vi "Convert to TDMS.vi"(6 "Fiirst call":bool, 8 "Error In":errorcluster, 9 "Add to channel list":string, 10 "TDMS target file":path, 11 "DataPlugin source file":path) -> (0 "Error Out":errorcluster, 1 "channel name(s) out":string[](array[string]), 2 "group name out":string, 3 "File output":path)   [LabVIEW 2015]
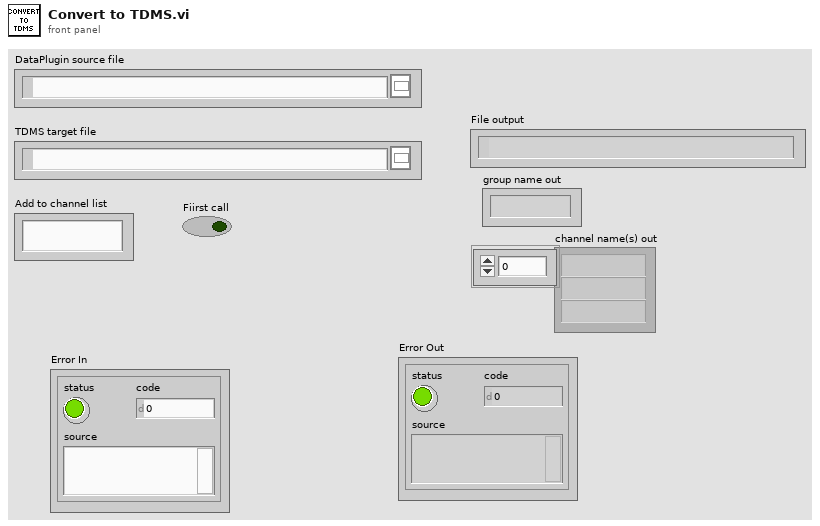
[diagram p1: front panel]
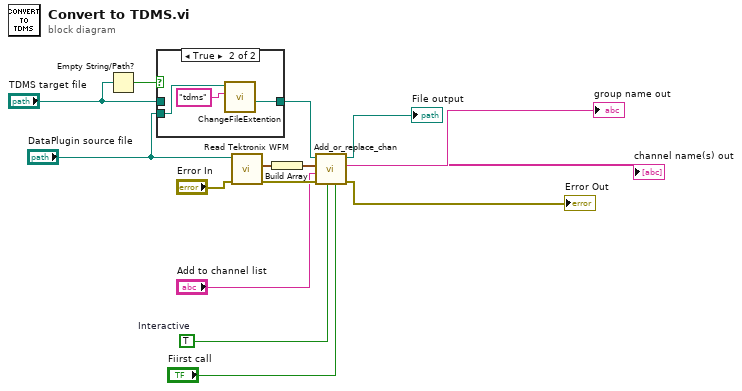
[diagram p0: block diagram]
diagram:
  w8 = TRUE  # Interactive
  n1 = Empty String/Path?(string/path="TDMS target file") -> (empty?=w11:bool)
  n2 = case shown="True" w11 {
    tunnel: "DataPlugin source file" -> [_ w18]
    tunnel: [w16 w17] -> w10
    tunnel: "TDMS target file" -> [w16 _]
    frame False {
    }
    frame True {
      n3 = call "ChangeFileExtention.vi"("New Extention"="tdms", "Path"=w18) -> ("Path with new extension"=w17:path)  [unwired: 5 in, 4 out]
    }
  }
  n4 = call "Read Tektronix WFM.vi"("Error In"="Error In", "WFM file Path"="DataPlugin source file") -> ("Error Out"=w13:errorcluster, "Waveform out"=w5:waveform(dbl))  [unwired: 7 in, 1 out]
  n5 = Build Array(w5) -> (w4:waveform(dbl)[])
  n6 = call "Add_or_replace_chan.vi"("Fiirst call"="Fiirst call", "Interactive"=w8, "Error In"=w13, "Add to channel list"="Add to channel list", "Waveforms"=w4, "File Path Control"=w10) -> ("Error Out"=→"Error Out":errorcluster, "channel name(s) out"=→"channel name(s) out":string[], "group name out"=→"group name out":string, "file path out"=→"File output":path)  [unwired: 2 in]
